vi "Seg2XY.vi"(8 "Length":i32, 9 "Layer":i32, 10 "List/Poly":bool, 11 "List":T1(array[cluster])) -> (3 "XY Graph":cluster{cluster{"X":sgl, "Y":sgl}[]}[](graph))   [LabVIEW 2014]
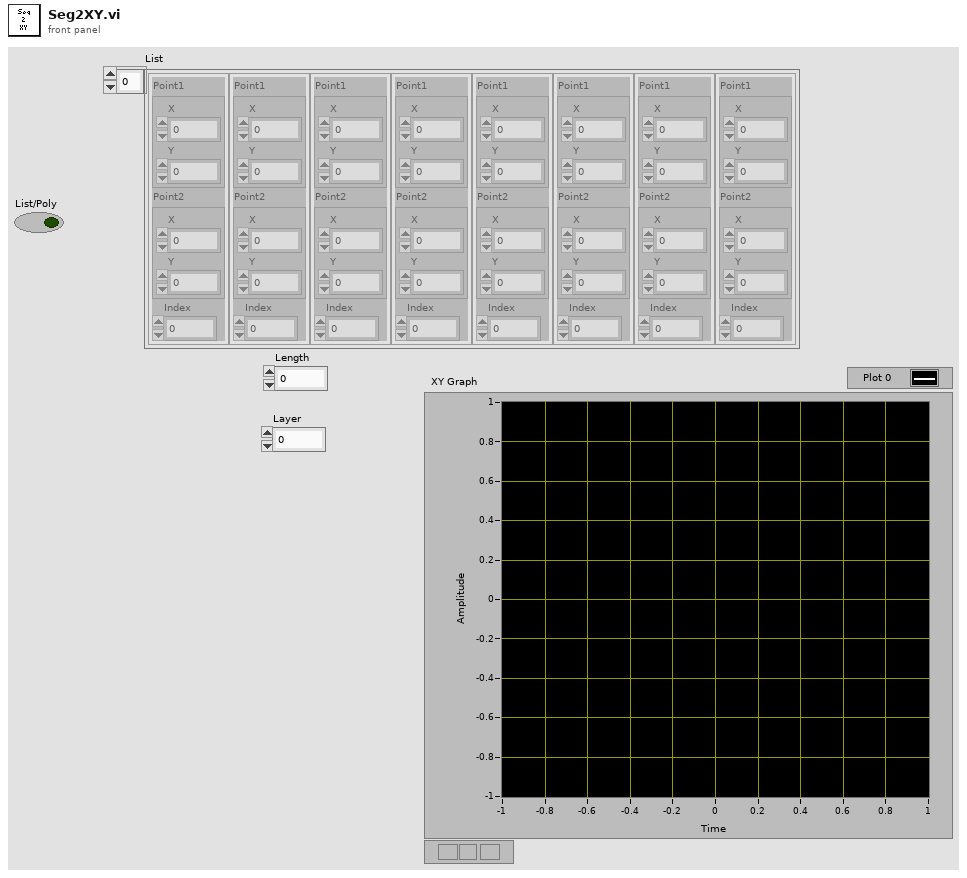
[diagram p1: front panel]
types:
  T1 = cluster{"Point1":cluster{"X":sgl, "Y":sgl}, "Point2":cluster{"X":sgl, "Y":sgl}, "Index":i32}[]
  T2 = cluster{"Point1":cluster{"X":sgl, "Y":sgl}, "Point2":cluster{"X":sgl, "Y":sgl}, "Index":i32}
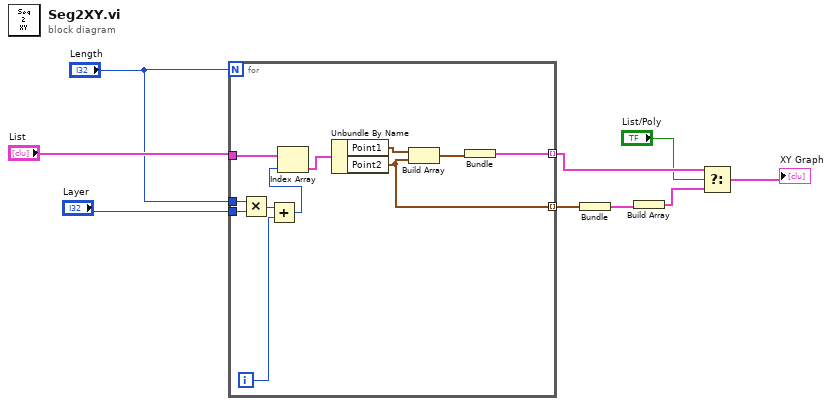
[diagram p0: block diagram]
diagram:
  n1 = for {
    N: "Length" -> [_]
    tunnel: "List" -> [w17]
    tunnel: [w18] -> w5 mode=indexing
    tunnel: "Layer" -> [w16]
    tunnel: "Length" -> [w15]
    tunnel: [w10] -> w6 mode=indexing
    i -> [w13]
    n2 = Multiply(x=w15, y=w16) -> (x*y=w14:i32)
    n3 = Add(x=w14, y=w13) -> (x+y=w12:i32)
    n4 = Index Array(array=w17, index=w12) -> (element=w11:T2)
    n5 = Unbundle By Name(w11) -> ("Point1"=w20:cluster{"X":sgl, "Y":sgl}, "Point2"=w10:cluster{"X":sgl, "Y":sgl})
    n6 = Build Array(w20, w10) -> (w19:cluster{"X":sgl, "Y":sgl}[])
    n7 = Bundle(w19) -> (w18:cluster{cluster{"X":sgl, "Y":sgl}[]})  [unwired: 1 in]
  }
  n8 = Bundle(w6) -> (w3:cluster{cluster{"X":sgl, "Y":sgl}[]})  [unwired: 1 in]
  n9 = Build Array(w3) -> (w2:cluster{cluster{"X":sgl, "Y":sgl}[]}[])
  n10 = Select(t=w5, s="List/Poly", f=w2) -> (s? t:f=→"XY Graph":cluster{cluster{"X":sgl, "Y":sgl}[]}[])
